vi "Stereo - Overlay Horizontal Lines.vi"(8 "error in (no error)":errorcluster, 10 "Interval":dbl=40.0, 11 "Rectified Image in":T1) -> (0 "error out":errorcluster, 3 "Rectified Image out":T1)   [LabVIEW 2017]
doc: "Overlay Horizontal lines onto the rectified images."
uses:
  <vilib>/vision/Image Controls.llb/IMAQ Image.ctl
panel:
  # "Overview: Overlay Horizontal lines onto the rectified images."
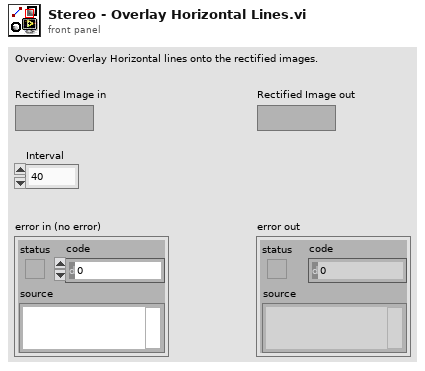
[diagram p1: front panel]
types:
  T1 = typedef "IMAQ Image.ctl" = refnum<image>
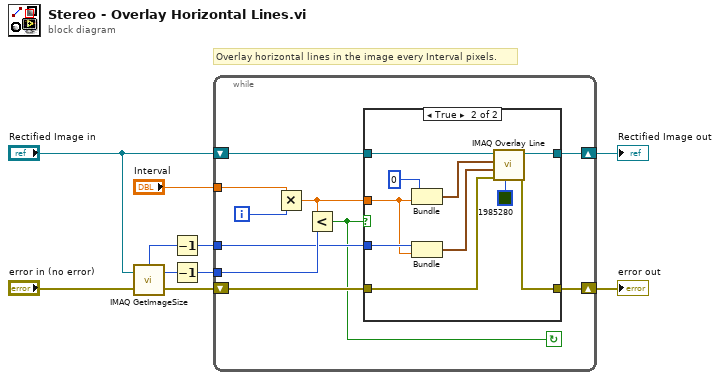
[diagram p0: block diagram]
diagram:
  # "Overlay horizontal lines in the image every Interval pixels."
  n1 = call "IMAQ GetImageSize"("Image"="Rectified Image in", "error in (no error)"="error in (no error)") -> ("Y Resolution"=w10:i32, "X Resolution"=w8:i32, "error out"=w6:errorcluster)  [unwired: 2 out]
  n2 = Decrement(x=w8) -> (x-1=w7:i32)
  n3 = Decrement(x=w10) -> (x-1=w9:i32)
  n4 = while {
    tunnel: w9 -> [w19]
    tunnel: w7 -> [w16]
    shift-right: [w14] -> w4
    shift-left: w6 -> [w15]
    shift-right: [w13] -> w5
    shift-left: "Rectified Image in" -> [w18]
    tunnel: "Interval" -> [w11]
    i -> [w20]
    stop <- w12 continue-if-true
    n5 = Multiply(x=w11, y=w20) -> (x*y=w17:dbl)
    n6 = Less?(x=w17, y=w19) -> (x < y?=w12:bool)
    n7 = case shown="True" w12 {
      tunnel: w18 -> [w22 w32]
      tunnel: w17 -> [_ w28]
      tunnel: w16 -> [_ w29]
      tunnel: w15 -> [w21 w26]
      tunnel: [w21 w25] -> w14
      tunnel: [w22 w24] -> w13
      frame False {
      }
      frame True {
        n8 = Bundle("X"=0, w28) -> (w30:cluster{"X":i32, dbl})  [unwired: 1 out]
        n9 = Bundle(w29, w28) -> (w27:cluster{i32, dbl})  [unwired: 1 out]
        n10 = call "IMAQ Overlay Line"("Color"=u32 1985280, "error in (no error)"=w26, "End Point"=w27, "Start Point"=w30, "Image"=w32) -> ("error out"=w25:errorcluster, "Image Out"=w24:T1)  [unwired: 1 in, 4 out]
      }
    }
  }
  "Rectified Image out" <- w5
  "error out" <- w4
